vi "print metal-CV.vi"() -> ()   [LabVIEW 2020]
panel:
  in  "Trigger B":bool
  in  "Voltage Step B (V)":dbl
  in  "Trigger A":bool
  in  "Voltage Step A (V)":dbl
  in  "Start":bool
  in  "停止":bool
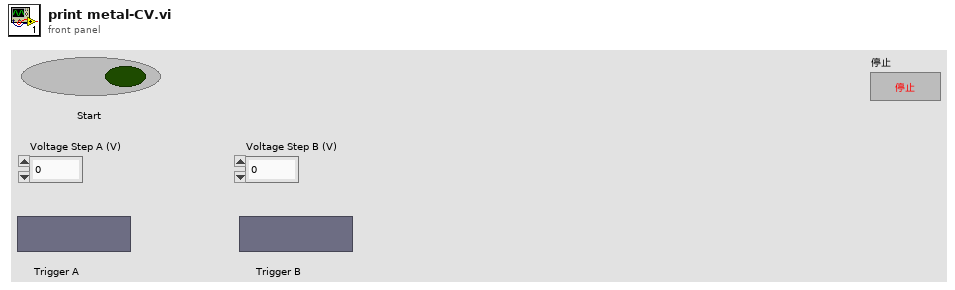
[diagram p1: front panel]
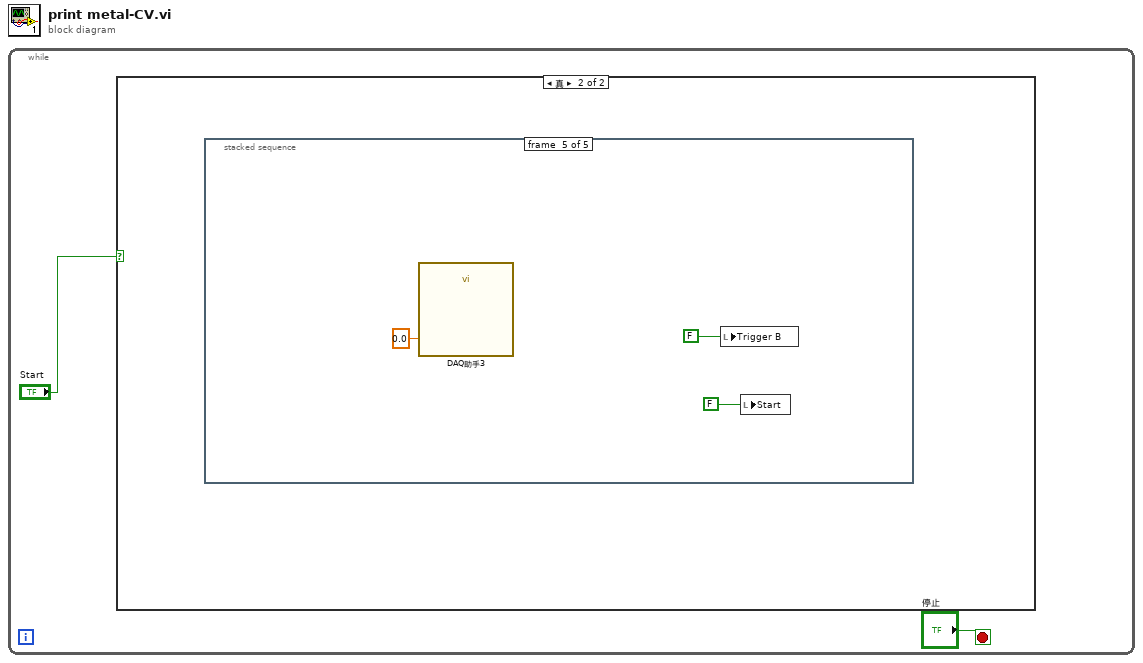
[diagram p0: block diagram]
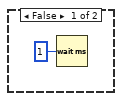
[diagram p2: hidden frame]
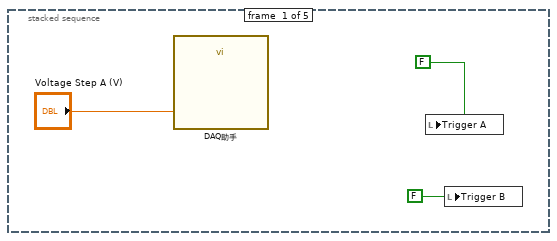
[diagram p3: hidden frame]
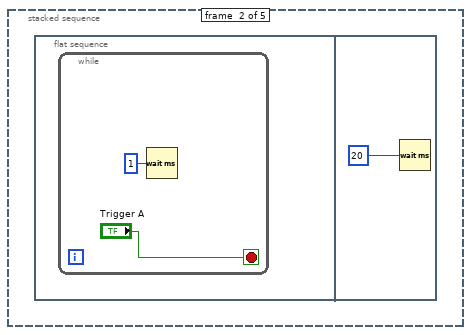
[diagram p4: hidden frame]
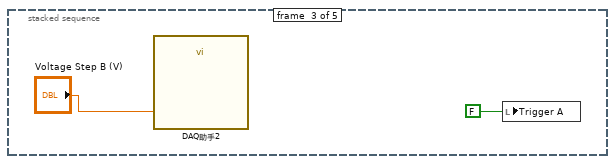
[diagram p5: hidden frame]
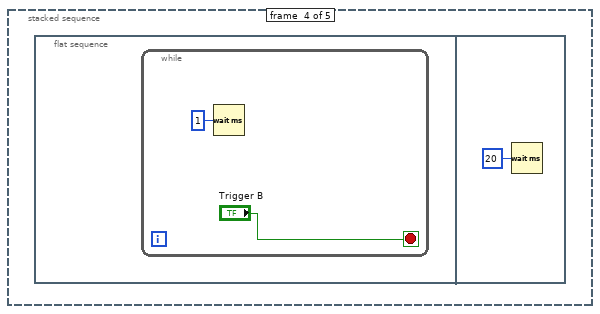
[diagram p6: hidden frame]
diagram:
  n1 = while {
    stop <- "停止" stop-if-true
    n2 = case shown="真" "Start" {
      frame False {
        n3 = Wait (ms)(milliseconds to wait=u32 1 ("等待时间（毫秒）")) -> ()  [unwired: 1 out]
      }
      frame True {
        n4 = stacked-sequence {
          frame #0 {
            n5 = call "DAQ助手"("data"="Voltage Step A (V)") -> ()  [unwired: 17 in, 2 out]
            n6 = local write "Trigger A"(FALSE) -> ()
            n7 = local write "Trigger B"(FALSE ("Trigger B")) -> ()
          }
          frame #1 {
            n8 = flat-sequence {
              frame #0 {
                n9 = while {
                  stop <- "Trigger A" stop-if-true
                  n10 = Wait (ms)(milliseconds to wait=u32 1 ("等待时间（毫秒）")) -> ()  [unwired: 1 out]
                }
              }
              frame #1 {
                n11 = Wait (ms)(milliseconds to wait=u32 20 ("等待时间（毫秒）")) -> ()  [unwired: 1 out]
              }
            }
          }
          frame #2 {
            n12 = call "DAQ助手2"("data"="Voltage Step B (V)") -> ()  [unwired: 17 in, 2 out]
            n13 = local write "Trigger A"(FALSE ("Trigger A")) -> ()
          }
          frame #3 {
            n14 = flat-sequence {
              frame #0 {
                n15 = while {
                  stop <- "Trigger B" stop-if-true
                  n16 = Wait (ms)(milliseconds to wait=u32 1 ("等待时间（毫秒）")) -> ()  [unwired: 1 out]
                }
              }
              frame #1 {
                n17 = Wait (ms)(milliseconds to wait=u32 20 ("等待时间（毫秒）")) -> ()  [unwired: 1 out]
              }
            }
          }
          frame #4 {
            n18 = call "DAQ助手3"("data"=0.0) -> ()  [unwired: 17 in, 2 out]
            n19 = local write "Trigger B"(FALSE ("Trigger B")) -> ()
            n20 = local write "Start"(FALSE ("Start")) -> ()
          }
        }
      }
    }
  }
